vi "Test 1.vi"() -> ()   [LabVIEW 2014]
panel:
  in  "Expect Response?":bool
  in  "VISA resource name":refnum<visa-resource-name>
  out "read buffer":string
  out "error out":errorcluster
  in  "write buffer":string
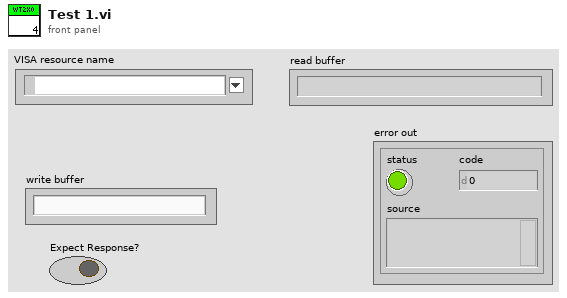
[diagram p1: front panel]
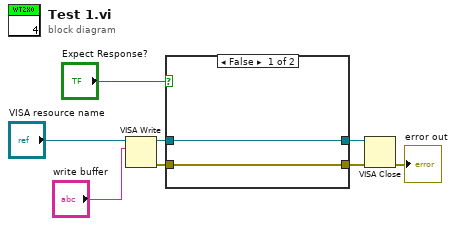
[diagram p0: block diagram]
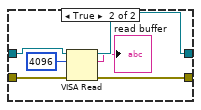
[diagram p2: hidden frame]
diagram:
  n1 = VISA Write(VISA resource name="VISA resource name", write buffer="write buffer") -> (VISA resource name out=w8:refnum<visa-resource-name>, error out=w7:errorcluster)  [unwired: 1 in, 1 out]
  n2 = case shown="False" "Expect Response?" {
    tunnel: w8 -> [w10 w16]
    tunnel: w7 -> [w9 w15]
    tunnel: [w10 w13] -> w5
    tunnel: [w9 w12] -> w4
    frame False {
    }
    frame True {
      n3 = VISA Read(VISA resource name=w16, byte count=u32 4096, error in (no error)=w15) -> (VISA resource name out=w13:refnum<visa-resource-name>, read buffer=→"read buffer":string, error out=w12:errorcluster)  [unwired: 1 out]
    }
  }
  n4 = VISA Close(VISA resource name=w5, error in (no error)=w4) -> (error out=→"error out":errorcluster)
